vi "pl1000Run.vi"(6 "method":enum16{"BM_SINGLE", "BM_WINDOW", "BM_STREAM"}(ring), 8 "error in (no error)":errorcluster, 10 "noOfValues":u16, 11 "pl1000 handle":i16) -> (0 "error out":errorcluster, 3 "pl1000 handle out":i16)   [LabVIEW 2016, in "pl1000.lvlib"]
doc: "This function tells the unit to start capturing data\n\nno_of_values: the total number of samples to be collected across all channels\n\nmethod: which method to use to collect the data, from the following list:\nBM_SINGLE\nBM_WINDOW\nBM_STREAM"
uses:
  pl1000.lvlib
  pl1000.dll
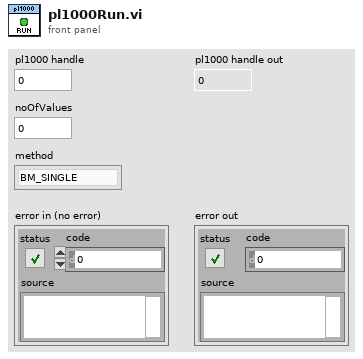
[diagram p1: front panel]
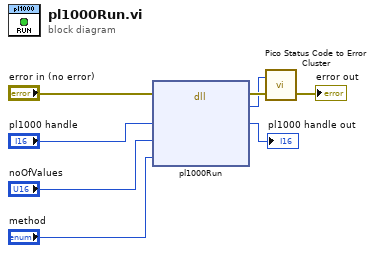
[diagram p0: block diagram]
diagram:
  n1 = dll-call lib="pl1000.dll" fn="pl1000Run"(error in="error in (no error)", "handle"="pl1000 handle", "noOfValues"="noOfValues", "method"="method") -> (error out=w6:errorcluster, "status"=w5:u32, "handle"=→"pl1000 handle out":i16)  [unwired: 4 in, 1 out]
  n2 = call "Pico Status Code to Error Cluster.vi"("error in"=w6, "PICO_STATUS"=w5) -> ("error out"=→"error out":errorcluster)  [unwired: 1 in]
